vi "WSVCAP SHL Host LL Set Write Data Parameter.vi"(0 "Write Byte In":u64, 11 "error in (no error)":errorcluster, 14 "FPGA":T1) -> (15 "error out":errorcluster)   [LabVIEW 2017]
uses:
  Type Defs/WSVCAP SHL FPGA Enum.ctl
  Type Defs/WSVCAP SHL Top Level Control Operation Enum.ctl
  Type Defs/WSVCAP SHL Top Level Control Enum.ctl
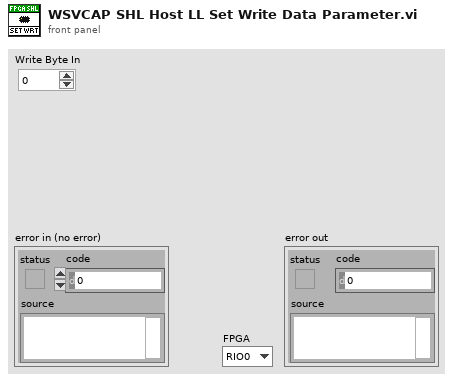
[diagram p1: front panel]
types:
  T1 = typedef "WSVCAP SHL FPGA Enum.ctl" = enum16{"RIO0", "RIO1"}
  T2 = typedef "WSVCAP SHL Top Level Control Enum.ctl" = enum16{"Start", "Cmd", "Transaction", "Wait Ticks", "Socket Mask", "UUT Set", "Slave Address", "Sub Address", "Bytes to Write", "Bytes to Read", "Write Data", "Write Flag", "Read Data", "Read Flag", "Ack Read", "Read Status Flag", "Ack Read Status", "Status", "Cycle Count", "Stop Cycle", "Exit"}
  T3 = typedef "WSVCAP SHL Top Level Control Operation Enum.ctl" = enum16{"Initialize", "Set Control", "Read Control", "Close"}
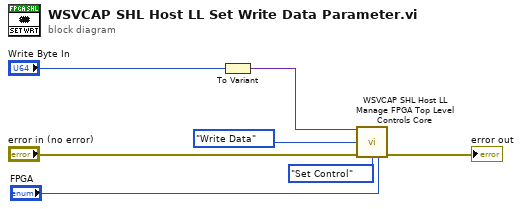
[diagram p0: block diagram]
diagram:
  n1 = To Variant(anything="Write Byte In") -> (Variant=w3:variant)
  n2 = call "WSVCAP SHL Host LL Manage FPGA Top Level Controls Core.vi"("Value In"=w3, "FPGA Top Level Control"=WSVCAP_SHL_Top_Level_Control_Enum."Write Data", "error in (no error)"="error in (no error)", "Operation"=WSVCAP_SHL_Top_Level_Control_Operation_Enum."Set Control", "FPGA"="FPGA") -> ("error out"=→"error out":errorcluster)  [unwired: 9 in, 1 out]
